vi "2Complement.vi"() -> ()   [LabVIEW 2017]
panel:
  out "Decimal":i32
  in  "12 bit":bool[](array[boolean])
  # "LSB"
  # "MSB"
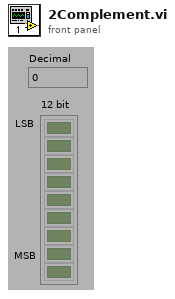
[diagram p1: front panel]
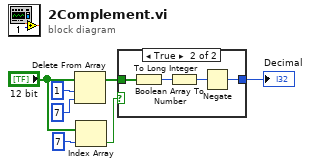
[diagram p0: block diagram]
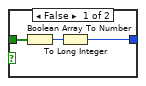
[diagram p2: hidden frame]
diagram:
  n1 = Delete From Array(array="12 bit", length=1, index=7) -> (array with subset deleted=w2:bool[])  [unwired: 1 out]
  n2 = Index Array(array="12 bit", index=7) -> (element=w6:bool)
  n3 = case shown="True" w6 {
    tunnel: w2 -> [w9 w13]
    tunnel: [w8 w11] -> w1
    frame False {
      n4 = Boolean Array To Number(Boolean array=w9) -> (number=w10:u32)
      n5 = To Long Integer(number=w10) -> (32bit integer=w8:i32)
    }
    frame True {
      n6 = Boolean Array To Number(Boolean array=w13) -> (number=w14:u32)
      n7 = To Long Integer(number=w14) -> (32bit integer=w12:i32)
      n8 = Negate(x=w12) -> (-x=w11:i32)
    }
  }
  "Decimal" <- w1
